vi "shift Register.vi"() -> ()   [LabVIEW 2022 SP3]
panel:
  out "Sequentiolly Grater":bool
  out "Previous Number":dbl
  in  "stop":bool
  out "number (0 to 1)":dbl
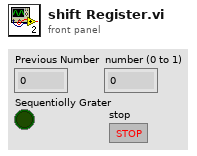
[diagram p1: front panel]
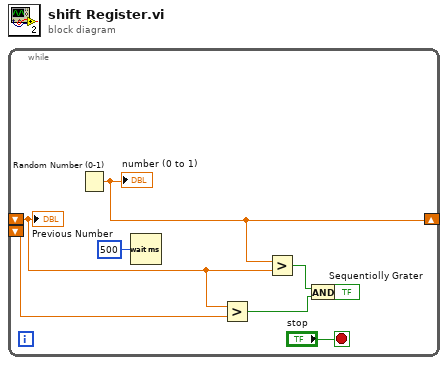
[diagram p0: block diagram]
diagram:
  n1 = while {
    shift-right: [w6] -> _
    shift-left: _ -> [w5]
    shift-left: _ -> [w4]
    stop <- "stop" stop-if-true
    n2 = Random Number (0-1)() -> (number: 0 to 1=w6:dbl)
    "number (0 to 1)" <- w6
    n3 = Wait (ms)(milliseconds to wait=u32 500) -> ()  [unwired: 1 out]
    n4 = Greater?(x=w5, y=w4) -> (0:w2:bool)
    n5 = Greater?(x=w6, y=w5) -> (0:w3:bool)
    n6 = And(x=w3, y=w2) -> (x .and. y?=→"Sequentiolly Grater":bool)
    "Previous Number" <- w5
  }
